vi "myRIO_BRig_Host_parse_dataTrial__v2.vi"(11 "arrayIn_dataTrial":u16[][](array[numeric])) -> (2 "appended array":cluster{i32[], i32[]}[](array[cluster]))   [LabVIEW 2014]
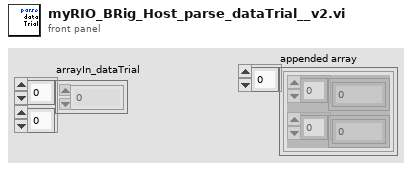
[diagram p1: front panel]
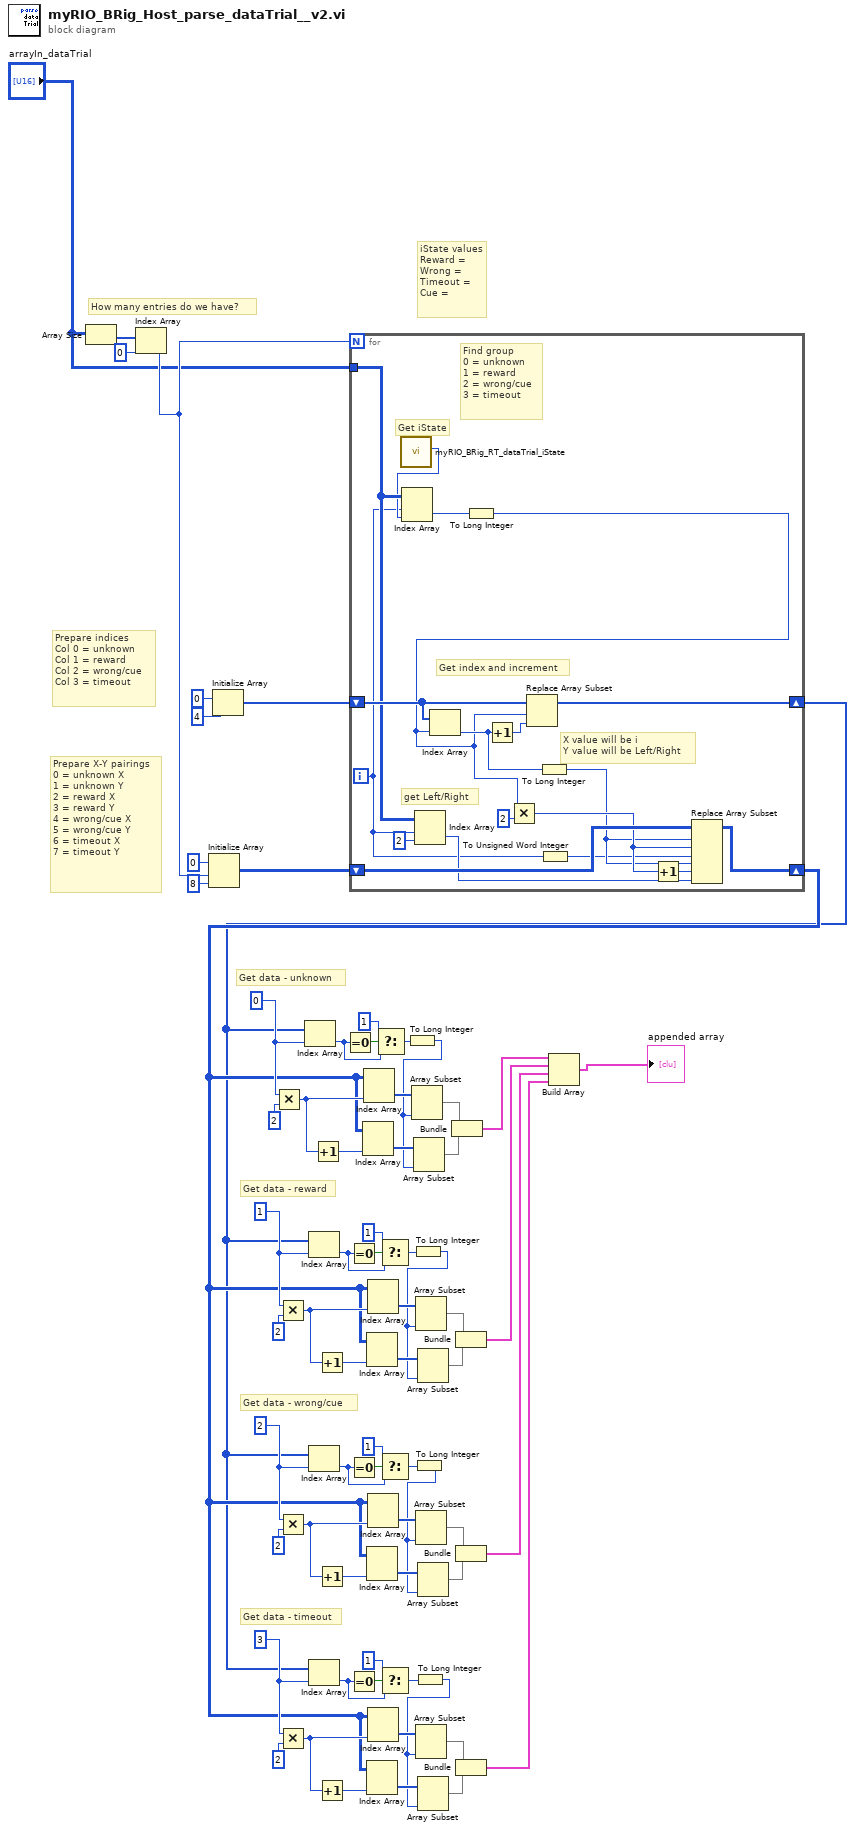
[diagram p0: block diagram]
diagram:
  w22 = 3 ("index")
  w33 = 2 ("index")
  w44 = 1 ("index")
  w55 = 0 ("index")
  # "Get data - timeout"
  # "Get data - wrong/cue"
  # "Get data - reward"
  # "Get data - unknown"
  # "Prepare X-Y pairings\n0 = unknown X\n1 = unknown Y\n2 = reward X\n3 = reward Y\n4 = wrong/cue X\n5 = wrong/cue Y\n6 = timeout X\n7 = timeout Y"
  # "Prepare indices\nCol 0 = unknown\nCol 1 = reward\nCol 2 = wrong/cue\nCol 3 = timeout"
  # "How many entries do we have?"
  # "iState values\nReward =\nWrong = \nTimeout = \nCue ="
  n1 = Array Size(array="arrayIn_dataTrial") -> (size(s)=w69:i32[])
  n2 = Index Array(array=w69, index=0) -> (element=w11:i32)
  n3 = Initialize Array(u16 0 ("element"), w11, 8 ("dimension size")) -> (w63:u16[][])
  n4 = Initialize Array(u16 0 ("element"), 4 ("dimension size")) -> (w62:u16[])
  n5 = Multiply(x=w55, y=2 ("index")) -> (x*y=w56:i32)
  n6 = Multiply(x=w44, y=2 ("index")) -> (x*y=w45:i32)
  n7 = Multiply(x=w33, y=2 ("index")) -> (x*y=w34:i32)
  n8 = Multiply(x=w22, y=2 ("index")) -> (x*y=w23:i32)
  n9 = Increment(x=w56) -> (x+1=w58:i32)
  n10 = Increment(x=w45) -> (x+1=w47:i32)
  n11 = Increment(x=w34) -> (x+1=w36:i32)
  n12 = Increment(x=w23) -> (x+1=w25:i32)
  n13 = for {
    N: w11 -> [_]
    shift-right: [w82] -> w17
    shift-left: w63 -> [w83]
    shift-right: [w86] -> w16
    shift-left: w62 -> [w87]
    tunnel: "arrayIn_dataTrial" -> [w77]
    i -> [w73]
    # "get Left/Right"
    # "X value will be i\nY value will be Left/Right"
    # "Get index and increment"
    # "Find group\n0 = unknown\n1 = reward\n2 = wrong/cue\n3 = timeout"
    # "Get iState"
    n14 = call "myRIO_BRig_RT_dataTrial_iState.vi"() -> ("output_iState"=w76:i32)  [unwired: 11 in]
    n15 = Index Array(array=w77, index (row)=w73, index (col)=w76) -> (element=w71:u16)
    n16 = Index Array(array=w77, index (row)=w73, index (col)=2 ("disabled index (col)")) -> (element=w81:u16)
    n17 = To Long Integer(number=w71) -> (32bit integer=w70:i32)
    n18 = Index Array(array=w87, index=w70) -> (element=w75:u16)
    n19 = Increment(x=w75) -> (x+1=w85:u16)
    n20 = Multiply(x=w70, y=2) -> (x*y=w78:i32)
    n21 = Replace Array Subset(array=w87, new element=w85, index=w70) -> (w86:u16[])
    n22 = To Long Integer(number=w75) -> (32bit integer=w74:i32)
    n23 = To Unsigned Word Integer(number=w73) -> (unsigned 16bit integer=w72:u16)
    n24 = Increment(x=w78) -> (x+1=w79:i32)
    n25 = Replace Array Subset(array=w83, new element #1=w72, index (row) #1=w74, index (col) #1=w78, new element #2=w81, index (row) #2=w74, index (col) #2=w79) -> (w82:u16[][])
  }
  n26 = Index Array(array=w16, index=w55) -> (element=w60:u16)
  n27 = Index Array(array=w16, index=w44) -> (element=w49:u16)
  n28 = Index Array(array=w16, index=w33) -> (element=w38:u16)
  n29 = Index Array(array=w16, index=w22) -> (element=w27:u16)
  n30 = Equal To 0?(x=w60) -> (x = 0?=w61:bool)
  n31 = Equal To 0?(x=w49) -> (x = 0?=w50:bool)
  n32 = Equal To 0?(x=w38) -> (x = 0?=w39:bool)
  n33 = Equal To 0?(x=w27) -> (x = 0?=w28:bool)
  n34 = Index Array(array=w17, index (col)=w58) -> (element=w57:u16[])  [unwired: 1 in]
  n35 = Index Array(array=w17, index (col)=w56) -> (element=w53:u16[])  [unwired: 1 in]
  n36 = Index Array(array=w17, index (col)=w47) -> (element=w46:u16[])  [unwired: 1 in]
  n37 = Index Array(array=w17, index (col)=w36) -> (element=w35:u16[])  [unwired: 1 in]
  n38 = Index Array(array=w17, index (col)=w25) -> (element=w24:u16[])  [unwired: 1 in]
  n39 = Index Array(array=w17, index (col)=w45) -> (element=w42:u16[])  [unwired: 1 in]
  n40 = Index Array(array=w17, index (col)=w34) -> (element=w31:u16[])  [unwired: 1 in]
  n41 = Index Array(array=w17, index (col)=w23) -> (element=w20:u16[])  [unwired: 1 in]
  n42 = Select(t=u16 1, s=w61, f=w60) -> (s? t:f=w10:u16)
  n43 = Select(t=u16 1, s=w50, f=w49) -> (s? t:f=w8:u16)
  n44 = Select(t=u16 1, s=w39, f=w38) -> (s? t:f=w6:u16)
  n45 = Select(t=u16 1, s=w28, f=w27) -> (s? t:f=w4:u16)
  n46 = To Long Integer(number=w10) -> (32bit integer=w9:i32)
  n47 = Array Subset(array=w53, length=w9) -> (w52:u16[])  [unwired: 1 in]
  n48 = To Long Integer(number=w8) -> (32bit integer=w7:i32)
  n49 = Array Subset(array=w57, length=w9) -> (w51:u16[])  [unwired: 1 in]
  n50 = To Long Integer(number=w6) -> (32bit integer=w5:i32)
  n51 = To Long Integer(number=w4) -> (32bit integer=w3:i32)
  n52 = Array Subset(array=w42, length=w7) -> (w41:u16[])  [unwired: 1 in]
  n53 = Array Subset(array=w31, length=w5) -> (w30:u16[])  [unwired: 1 in]
  n54 = Array Subset(array=w20, length=w3) -> (w19:u16[])  [unwired: 1 in]
  n55 = Array Subset(array=w46, length=w7) -> (w40:u16[])  [unwired: 1 in]
  n56 = Array Subset(array=w35, length=w5) -> (w29:u16[])  [unwired: 1 in]
  n57 = Array Subset(array=w24, length=w3) -> (w18:u16[])  [unwired: 1 in]
  n58 = Bundle(w52, w51) -> (w15:cluster{u16[], u16[]})  [unwired: 1 in]
  n59 = Bundle(w41, w40) -> (w14:cluster{u16[], u16[]})  [unwired: 1 in]
  n60 = Bundle(w30, w29) -> (w13:cluster{u16[], u16[]})  [unwired: 1 in]
  n61 = Bundle(w19, w18) -> (w12:cluster{u16[], u16[]})  [unwired: 1 in]
  n62 = Build Array(w15, w14, w13, w12) -> (→"appended array":cluster{u16[], u16[]}[])
